vi "correct map.vi"(10 "Map dimensions":dbl[](array[numeric]), 11 "Obsticle map":u16[][](array[ring])) -> (3 "Corrected map":u16[][](array[ring]))   [LabVIEW 2015]
panel:
  out "y":dbl
  out "x":dbl
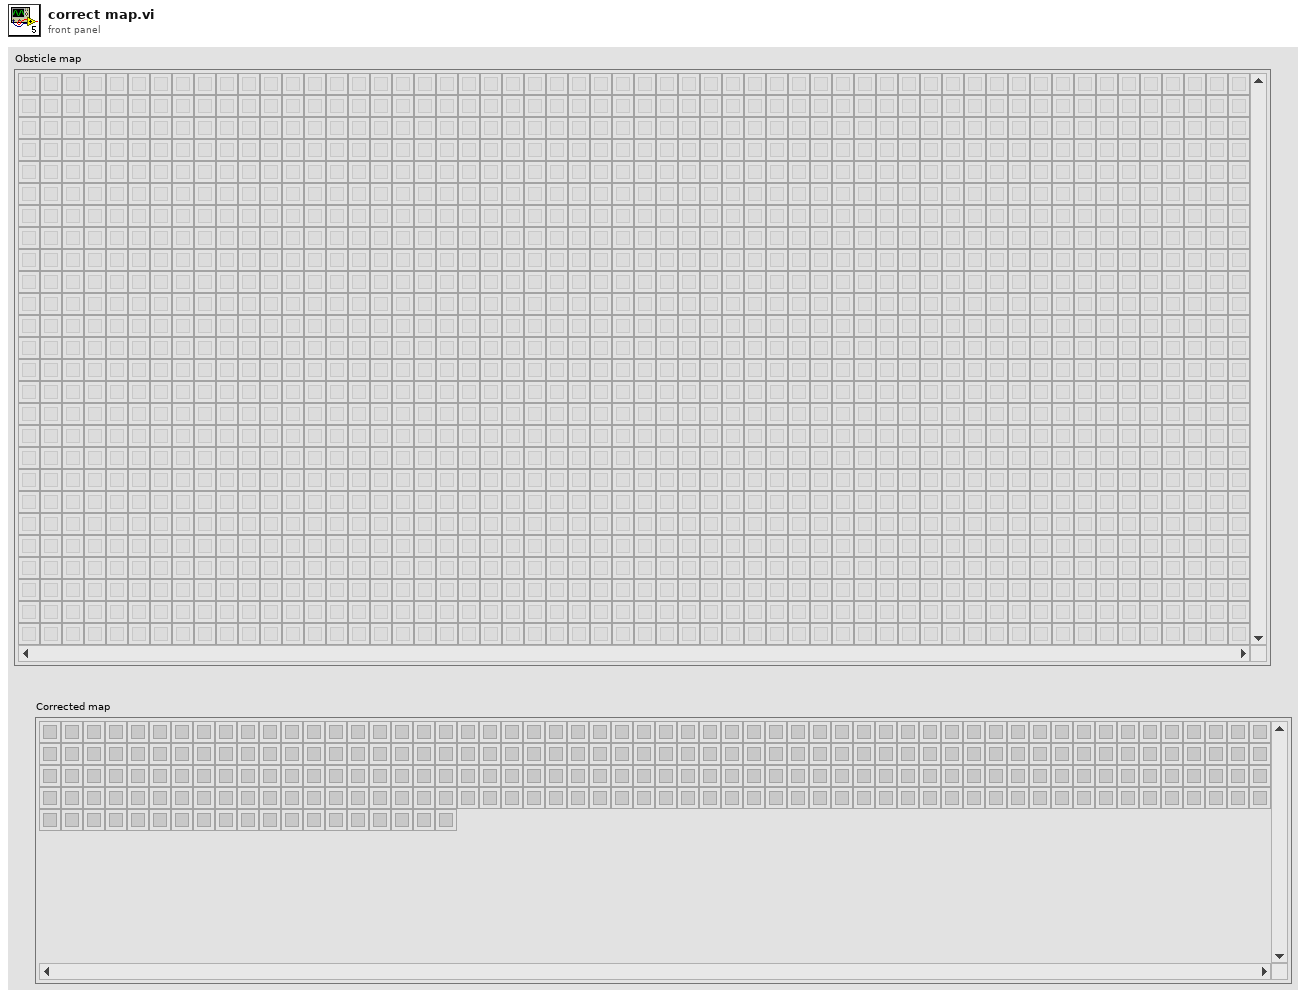
[diagram p1: front panel]
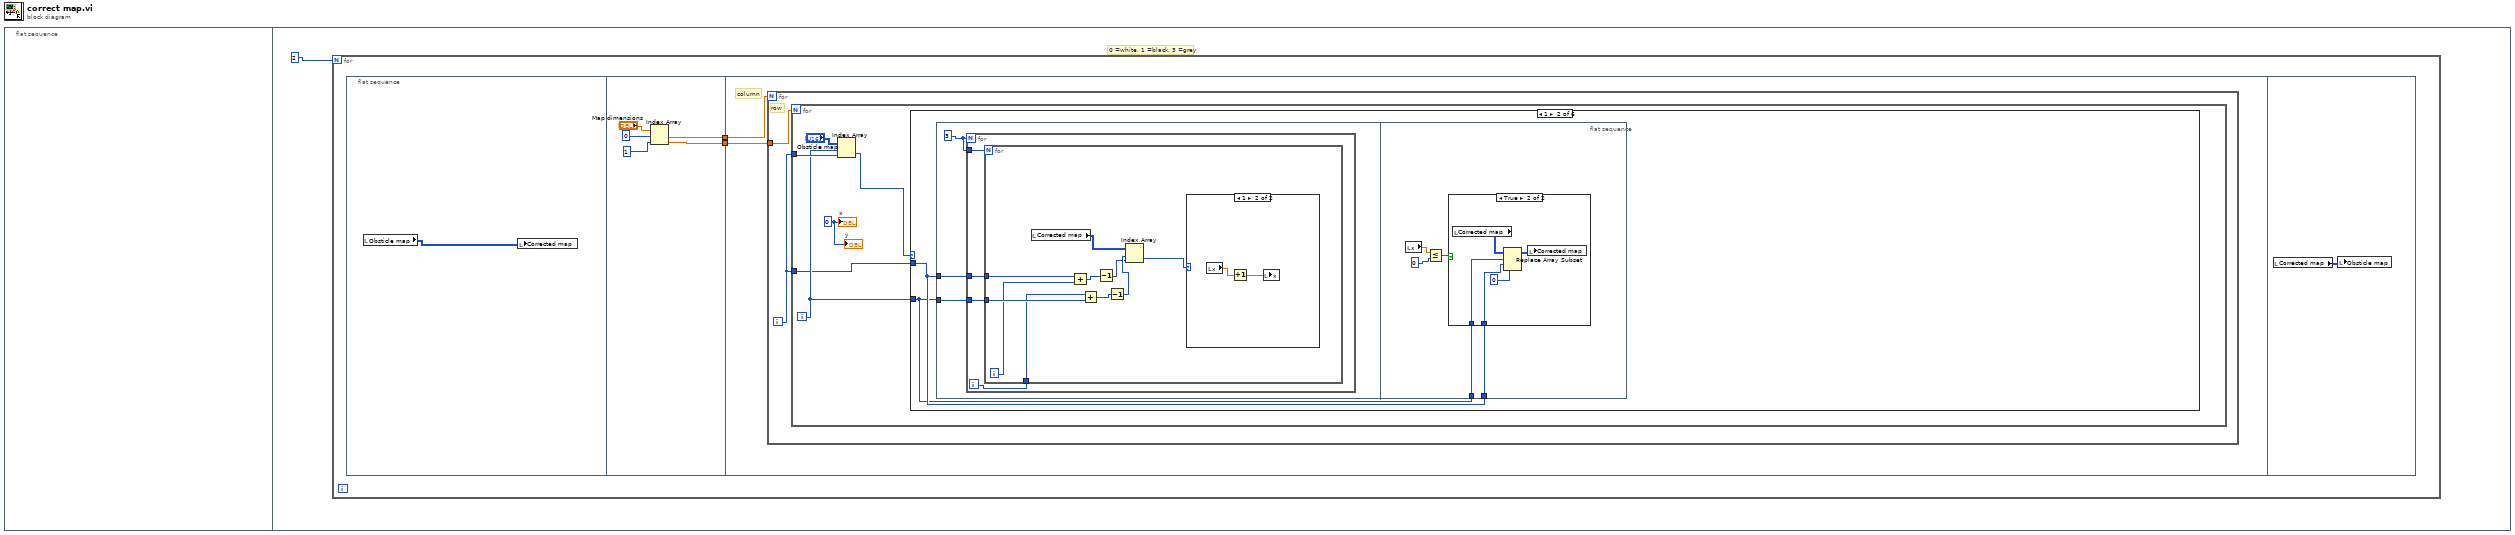
[diagram p0: block diagram]
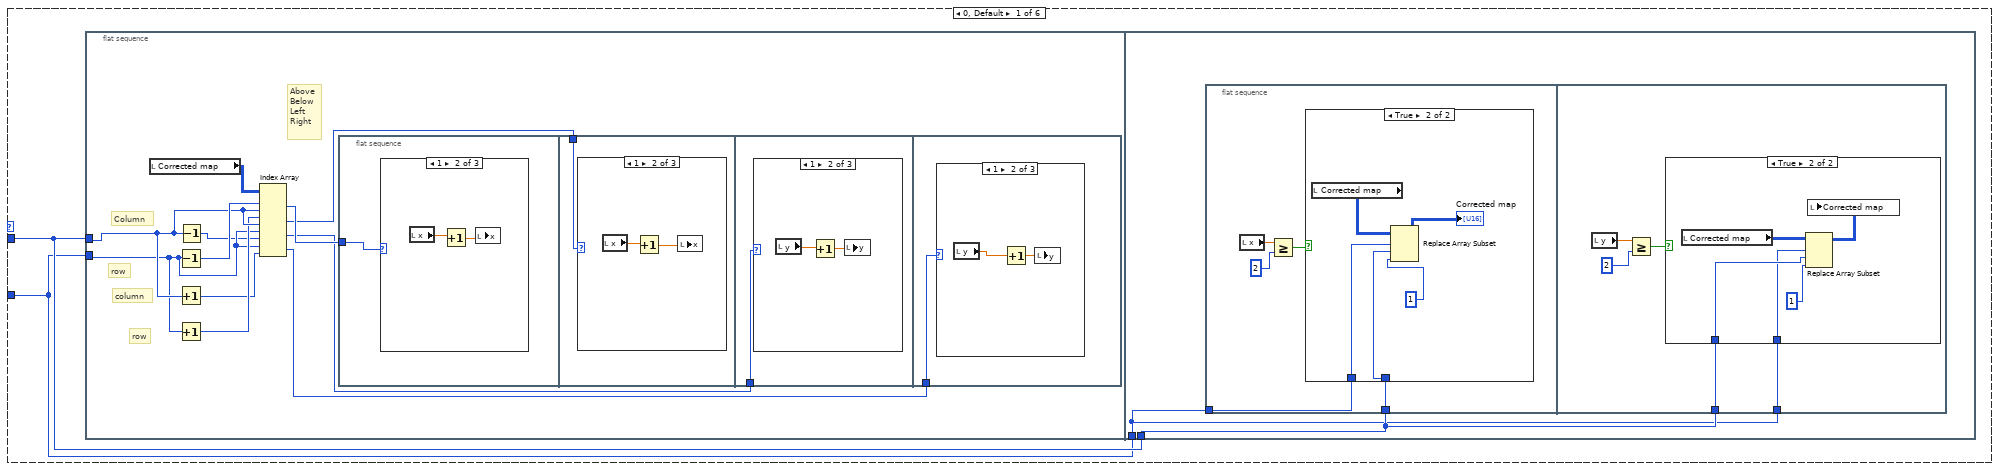
[diagram p2: hidden frame]
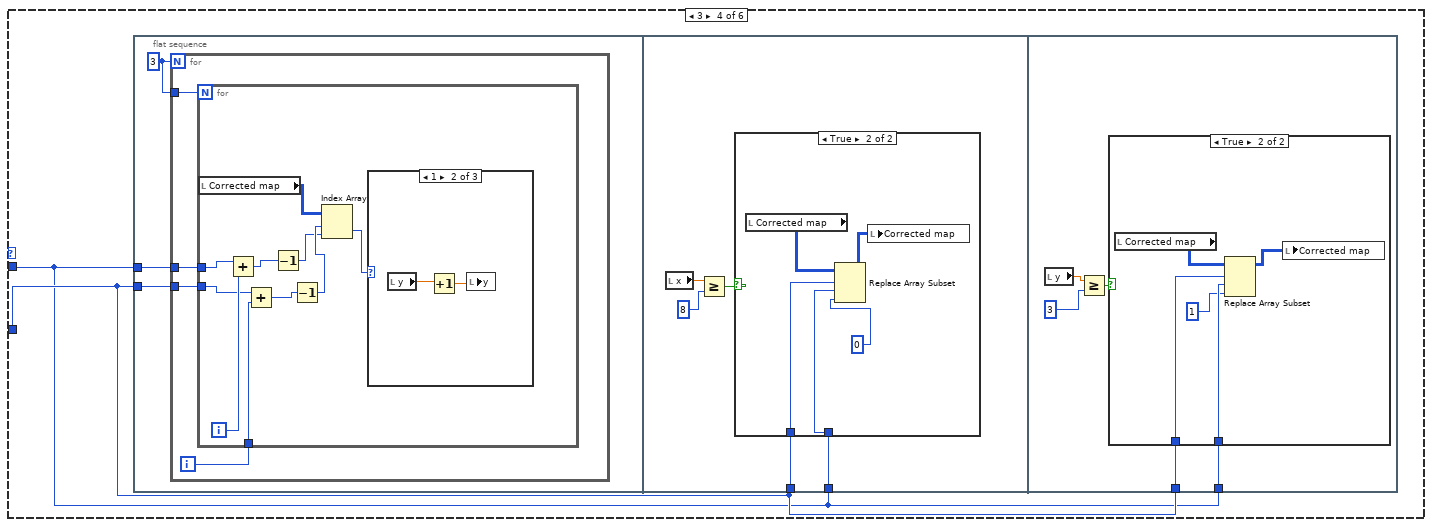
[diagram p16: hidden frame]
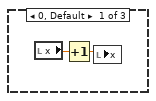
[diagram p17: hidden frame]
diagram:
  n1 = flat-sequence {
    frame #0 {
    }
    frame #1 {
      # "0 =white, 1 =black, 3 =grey"
      n2 = for {
        N: 2 -> [_]
        n3 = flat-sequence {
          tunnel: [w7] -> w3
          tunnel: [w6] -> w2
          tunnel: w3 -> [w11]
          tunnel: w2 -> [w10]
          frame #0 {
            n4 = local read "Obsticle map"() -> (w4:u16[][])
            n5 = local write "Corrected map"(w4) -> ()
          }
          frame #1 {
            n6 = Index Array(array="Map dimensions", index #1=0, index #2=1) -> (element #1=w7:dbl, element #2=w6:dbl)
          }
          frame #2 {
            # "column"
            n7 = for {
              N: w11 -> [_]
              tunnel: w10 -> [w13]
              i -> [w12]
              # "row"
              n8 = for {
                N: w13 -> [_]
                tunnel: w12 -> [w18]
                tunnel: w12 -> [w16]
                i -> [w17]
                w14 = 0
                n9 = Index Array(array="Obsticle map", index (row)=w17, index (col)=w18) -> (element=w15:u16)
                n10 = case shown="1" w15 {
                  tunnel: w17 -> [w20 w67 _ w99 _ _]
                  tunnel: w16 -> [w21 w68 _ w98 _ _]
                  frame 0, Default {
                    n11 = flat-sequence {
                      tunnel: w20 -> [w27]
                      tunnel: w21 -> [w29]
                      tunnel: w21 -> [w46]
                      tunnel: w20 -> [w45]
                      frame #0 {
                        # "Above\nBelow\nLeft\nRight"
                        # "row"
                        # "column"
                        # "row"
                        # "Column"
                        n12 = local read "Corrected map"() -> (w32:u16[][])
                        n13 = Decrement(x=w27) -> (x-1=w30:i32)
                        n14 = Increment(x=w29) -> (x+1=w26:i32)
                        n15 = Increment(x=w27) -> (x+1=w28:i32)
                        n16 = Decrement(x=w29) -> (x-1=w25:i32)
                        n17 = Index Array(array=w32, index (row) #1=w30, index (col) #1=w29, index (row) #2=w28, index (col) #2=w29, index (row) #3=w27, index (col) #3=w25, index (row) #4=w27, index (col) #4=w26) -> (element #1=w31:u16, element #2=w24:u16, element #3=w23:u16, element #4=w22:u16)
                        n18 = flat-sequence {
                          tunnel: w31 -> [w33]
                          tunnel: w24 -> [w36]
                          tunnel: w23 -> [w39]
                          tunnel: w22 -> [w42]
                          frame #0 {
                            n19 = case shown="1" w33 {
                              frame 0, Default {
                              }
                              frame 1 {
                                n20 = local read "x"() -> (w35:dbl)
                                n21 = Increment(x=w35) -> (x+1=w34:dbl)
                                n22 = local write "x"(w34) -> ()
                              }
                              frame 3 {
                              }
                            }
                          }
                          frame #1 {
                            n23 = case shown="1" w36 {
                              frame 0, Default {
                              }
                              frame 1 {
                                n24 = local read "x"() -> (w37:dbl)
                                n25 = Increment(x=w37) -> (x+1=w38:dbl)
                                n26 = local write "x"(w38) -> ()
                              }
                              frame 3 {
                              }
                            }
                          }
                          frame #2 {
                            n27 = case shown="1" w39 {
                              frame 0, Default {
                              }
                              frame 1 {
                                n28 = local read "y"() -> (w40:dbl)
                                n29 = Increment(x=w40) -> (x+1=w41:dbl)
                                n30 = local write "y"(w41) -> ()
                              }
                              frame 3 {
                              }
                            }
                          }
                          frame #3 {
                            n31 = case shown="1" w42 {
                              frame 0, Default {
                              }
                              frame 1 {
                                n32 = local read "y"() -> (w43:dbl)
                                n33 = Increment(x=w43) -> (x+1=w44:dbl)
                                n34 = local write "y"(w44) -> ()
                              }
                              frame 3 {
                              }
                            }
                          }
                        }
                      }
                      frame #1 {
                        n35 = flat-sequence {
                          tunnel: w45 -> [w48]
                          tunnel: w46 -> [w47]
                          tunnel: w46 -> [w58]
                          tunnel: w45 -> [w57]
                          frame #0 {
                            n36 = local read "x"() -> (w50:dbl)
                            n37 = Greater Or Equal?(x=w50, y=2) -> (x >= y?=w51:bool)
                            n38 = case shown="True" w51 {
                              tunnel: w47 -> [_ w55]
                              tunnel: w48 -> [_ w54]
                              frame False {
                              }
                              frame True {
                                n39 = local read "Corrected map"() -> (w56:u16[][])
                                n40 = Replace Array Subset(array=w56, new element=1, index (row)=w54, index (col)=w55) -> (→"Corrected map":u16[][])
                              }
                            }
                          }
                          frame #1 {
                            n41 = local read "y"() -> (w61:dbl)
                            n42 = Greater Or Equal?(x=w61, y=2) -> (x >= y?=w59:bool)
                            n43 = case shown="True" w59 {
                              tunnel: w58 -> [_ w63]
                              tunnel: w57 -> [_ w62]
                              frame False {
                              }
                              frame True {
                                n44 = local read "Corrected map"() -> (w65:u16[][])
                                n45 = Replace Array Subset(array=w65, new element=1, index (row)=w62, index (col)=w63) -> (w64:u16[][])
                                n46 = local write "Corrected map"(w64) -> ()
                              }
                            }
                          }
                        }
                      }
                    }
                  }
                  frame 1 {
                    n47 = flat-sequence {
                      tunnel: w68 -> [w69]
                      tunnel: w67 -> [w70]
                      tunnel: w68 -> [w89]
                      tunnel: w67 -> [w88]
                      frame #0 {
                        w71 = 3
                        n48 = for {
                          N: w71 -> [_]
                          tunnel: w71 -> [w75]
                          tunnel: w69 -> [w74]
                          tunnel: w70 -> [w73]
                          i -> [w72]
                          n49 = for {
                            N: w75 -> [_]
                            tunnel: w74 -> [w80]
                            tunnel: w73 -> [w79]
                            tunnel: w72 -> [w76]
                            i -> [w78]
                            n50 = local read "Corrected map"() -> (w77:u16[][])
                            n51 = Add(x=w80, y=w78) -> (x+y=w84:i32)
                            n52 = Add(x=w76, y=w79) -> (x+y=w85:i32)
                            n53 = Decrement(x=w84) -> (x-1=w82:i32)
                            n54 = Decrement(x=w85) -> (x-1=w83:i32)
                            n55 = Index Array(array=w77, index (row)=w83, index (col)=w82) -> (element=w81:u16)
                            n56 = case shown="1" w81 {
                              frame 0, Default {
                              }
                              frame 1 {
                                n57 = local read "x"() -> (w87:dbl)
                                n58 = Increment(x=w87) -> (x+1=w86:dbl)
                                n59 = local write "x"(w86) -> ()
                              }
                            }
                          }
                        }
                      }
                      frame #1 {
                        n60 = local read "x"() -> (w91:dbl)
                        n61 = Less Or Equal?(x=w91, y=0) -> (x <= y?=w92:bool)
                        n62 = case shown="True" w92 {
                          tunnel: w89 -> [_ w95]
                          tunnel: w88 -> [_ w94]
                          frame False {
                          }
                          frame True {
                            n63 = local read "Corrected map"() -> (w97:u16[][])
                            n64 = Replace Array Subset(array=w97, new element=0, index (row)=w94, index (col)=w95) -> (w96:u16[][])
                            n65 = local write "Corrected map"(w96) -> ()
                          }
                        }
                      }
                    }
                  }
                  frame 2 {
                  }
                  frame 3 {
                    n66 = flat-sequence {
                      tunnel: w99 -> [w101]
                      tunnel: w98 -> [w100]
                      tunnel: w98 -> [w122]
                      tunnel: w99 -> [w121]
                      tunnel: w99 -> [w135]
                      tunnel: w98 -> [w134]
                      frame #0 {
                        w102 = 3
                        n67 = for {
                          N: w102 -> [_]
                          tunnel: w102 -> [w106]
                          tunnel: w101 -> [w105]
                          tunnel: w100 -> [w104]
                          i -> [w103]
                          n68 = for {
                            N: w106 -> [_]
                            tunnel: w105 -> [w112]
                            tunnel: w104 -> [w115]
                            tunnel: w103 -> [w113]
                            i -> [w114]
                            n69 = local read "Corrected map"() -> (w116:u16[][])
                            n70 = Add(x=w115, y=w114) -> (x+y=w110:i32)
                            n71 = Add(x=w112, y=w113) -> (x+y=w111:i32)
                            n72 = Decrement(x=w110) -> (x-1=w107:i32)
                            n73 = Decrement(x=w111) -> (x-1=w108:i32)
                            n74 = Index Array(array=w116, index (row)=w108, index (col)=w107) -> (element=w109:u16)
                            n75 = case shown="1" w109 {
                              frame 0, Default {
                                n76 = local read "x"() -> (w117:dbl)
                                n77 = Increment(x=w117) -> (x+1=w118:dbl)
                                n78 = local write "x"(w118) -> ()
                              }
                              frame 1 {
                                n79 = local read "y"() -> (w120:dbl)
                                n80 = Increment(x=w120) -> (x+1=w119:dbl)
                                n81 = local write "y"(w119) -> ()
                              }
                              frame 3 {
                              }
                            }
                          }
                        }
                      }
                      frame #1 {
                        n82 = local read "x"() -> (w124:dbl)
                        n83 = Greater Or Equal?(x=w124, y=8) -> (x >= y?=w125:bool)
                        n84 = case shown="True" w125 {
                          tunnel: w122 -> [_ w128]
                          tunnel: w121 -> [_ w127]
                          frame False {
                          }
                          frame True {
                            n85 = local read "Corrected map"() -> (w130:u16[][])
                            n86 = Replace Array Subset(array=w130, new element=0, index (row)=w127, index (col)=w128) -> (w129:u16[][])
                            n87 = local write "Corrected map"(w129) -> ()
                          }
                        }
                      }
                      frame #2 {
                        n88 = local read "y"() -> (w132:dbl)
                        n89 = Greater Or Equal?(x=w132, y=3) -> (x >= y?=w133:bool)
                        n90 = case shown="True" w133 {
                          tunnel: w135 -> [_ w140]
                          tunnel: w134 -> [_ w139]
                          frame False {
                          }
                          frame True {
                            n91 = local read "Corrected map"() -> (w137:u16[][])
                            n92 = Replace Array Subset(array=w137, new element=1, index (row)=w140, index (col)=w139) -> (w138:u16[][])
                            n93 = local write "Corrected map"(w138) -> ()
                          }
                        }
                      }
                    }
                  }
                  frame 4 {
                  }
                  frame 5 {
                  }
                }
                "x" <- w14
                "y" <- w14
              }
            }
          }
          frame #3 {
            n94 = local read "Corrected map"() -> (w141:u16[][])
            n95 = local write "Obsticle map"(w141) -> ()
          }
        }
      }
    }
  }
